vi "_21_Sample_qsns_10[1].vi"() -> ()   [LabVIEW 2020]
panel:
  out "appended array":dbl[][](array[numeric])
  out "subarray":dbl[](array[numeric])
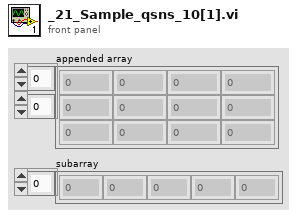
[diagram p1: front panel]
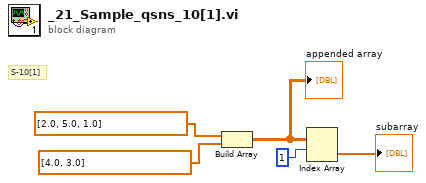
[diagram p0: block diagram]
diagram:
  # "S-10[1]"
  n1 = Build Array "Build Array"(dbl[] [2.0, 5.0, 1.0], dbl[] [4.0, 3.0]) -> (w3:dbl[][])
  "appended array" <- w3
  n2 = Index Array "Index Array"(array=w3, index (row)=1) -> (element=→"subarray":dbl[])  [unwired: 1 in]
